vi "Read Help File.vi"(8 "error in (no error)":errorcluster, 11 "MetaDataObj.lvclass":refnum<class "MetaDataObj.lvclass">) -> (0 "error out":errorcluster, 2 "Cluster":T1, 3 "MetaDataObj.lvclass out":refnum<class "MetaDataObj.lvclass">)   [LabVIEW 2016, in "MetaDataObj.lvclass"]
uses:
  <resource>/dialog/NewProjectWizard/MetaDataObj/MetaDataObj.lvclass
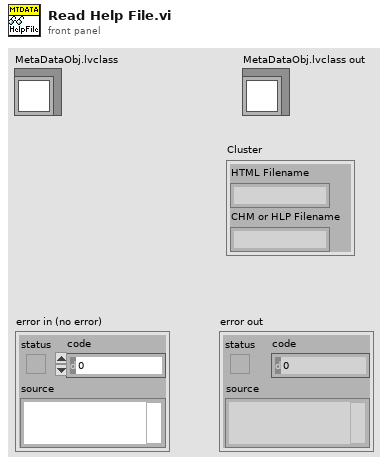
[diagram p1: front panel]
types:
  T1 = cluster{"HTML Filename":string, "CHM or HLP Filename":string}
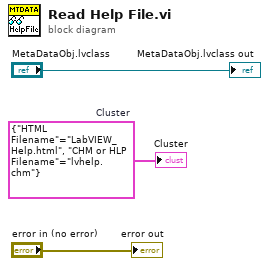
[diagram p0: block diagram]
diagram:
  w2 = T1 {"HTML Filename"="LabVIEW_Help.html", "CHM or HLP Filename"="lvhelp.chm"}  # Cluster
  "MetaDataObj.lvclass out" <- "MetaDataObj.lvclass"
  "error out" <- "error in (no error)"
  "Cluster" <- w2
